vi "ZApproachingPart.vi"() -> ()   [LabVIEW 2014]
uses:
  <vilib>/userdefined/High Color/nirio_resource_hc.ctl
  <vilib>/Instr/_visa.llb/VISA Configure Serial Port (Instr).vi
  <vilib>/FPGAPlugInAG/PCIe-7851R/niLvFpga_Open_PCIe-7851R.vi
  <vilib>/rvi/interface/common/dynamic/niFpgaDynamicAddResources.vi
  <vilib>/Utility/error.llb/Error Cluster From Error Code.vi
  <vilib>/rvi/errors/niLvFpgaAdjustHostInterfaceError.vi
  <vilib>/FPGAPlugInAG/Dynamic/niLvFpga_Close_Dynamic.vi
  <vilib>/rvi/interface/nirviOpenFPGA/nirviOpenFPGA.xnode
  FPGA Bitfiles/FPGATest_FPGATarget_PIZApproaching_ngy2QjQf4ns.lvbitx
  <vilib>/rvi/interface/nirviReadWriteControl/nirviReadWriteControl.xnode
  <vilib>/rvi/interface/nirviCloseFPGA/nirviCloseFPGA.xnode
  FPGA Bitfiles/FPGATest_FPGATarget_PIZWithdraw_iPHi2cM2eR0.lvbitx
  NiFpgaLv.dll
  <vilib>/rvi/interface/Simulation/niFpgaSimulationCallBeginRW.vi
panel:
  out "RoughXYZPosDia":dbl(graph)
  out "RoughXYZErr?":string
  in  "LandingPtRelativeToPIZ/um  Range(0-10)":dbl format="%#_13g"
  out "RoughZPos?":dbl format="%#_13g"
  out "MaxPIZPos":i16
  in  "PIZ":T1
  out "preCurrIndexDia":i16(graph)
  out "preCurrIndex":i16
  out "refCurrIndex":i16
  out "PIZPos":i16
  out "PIZPosDia":i16(graph)
  in  "stop":bool
  in  "AllLoopSleep ms":i32
  in  "thresholdIndex":i32
  in  "RoughXYZ":refnum<visa-resource-name>
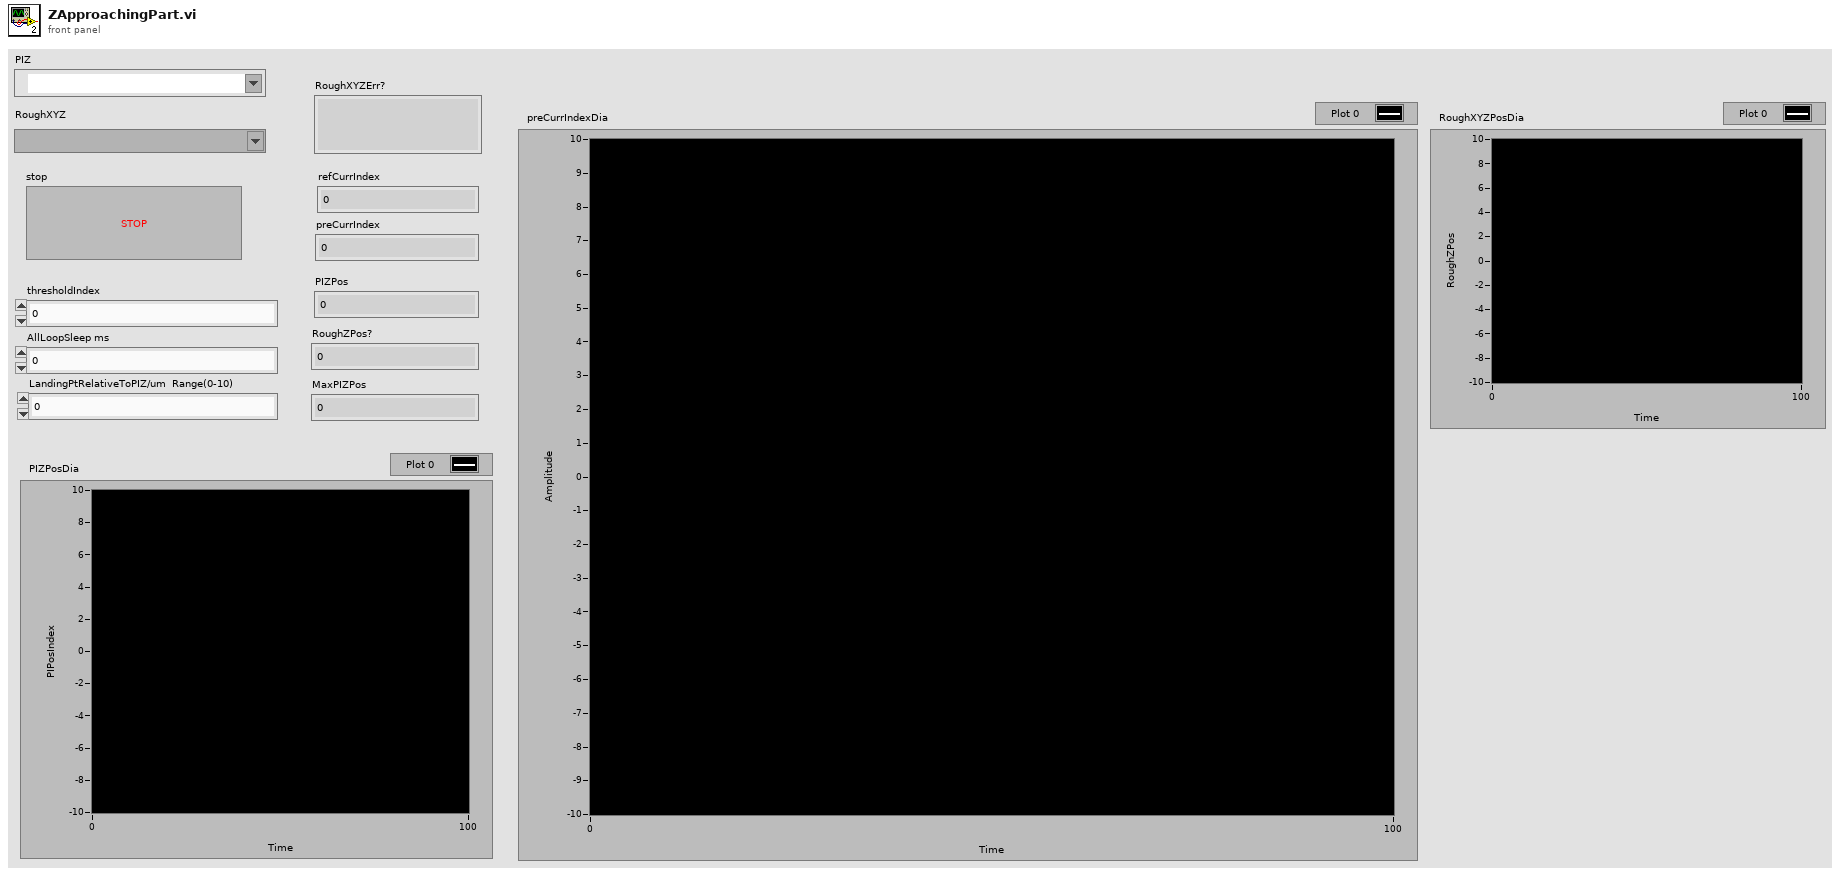
[diagram p1: front panel]
types:
  T1 = typedef "nirio_resource_hc.ctl" = tag
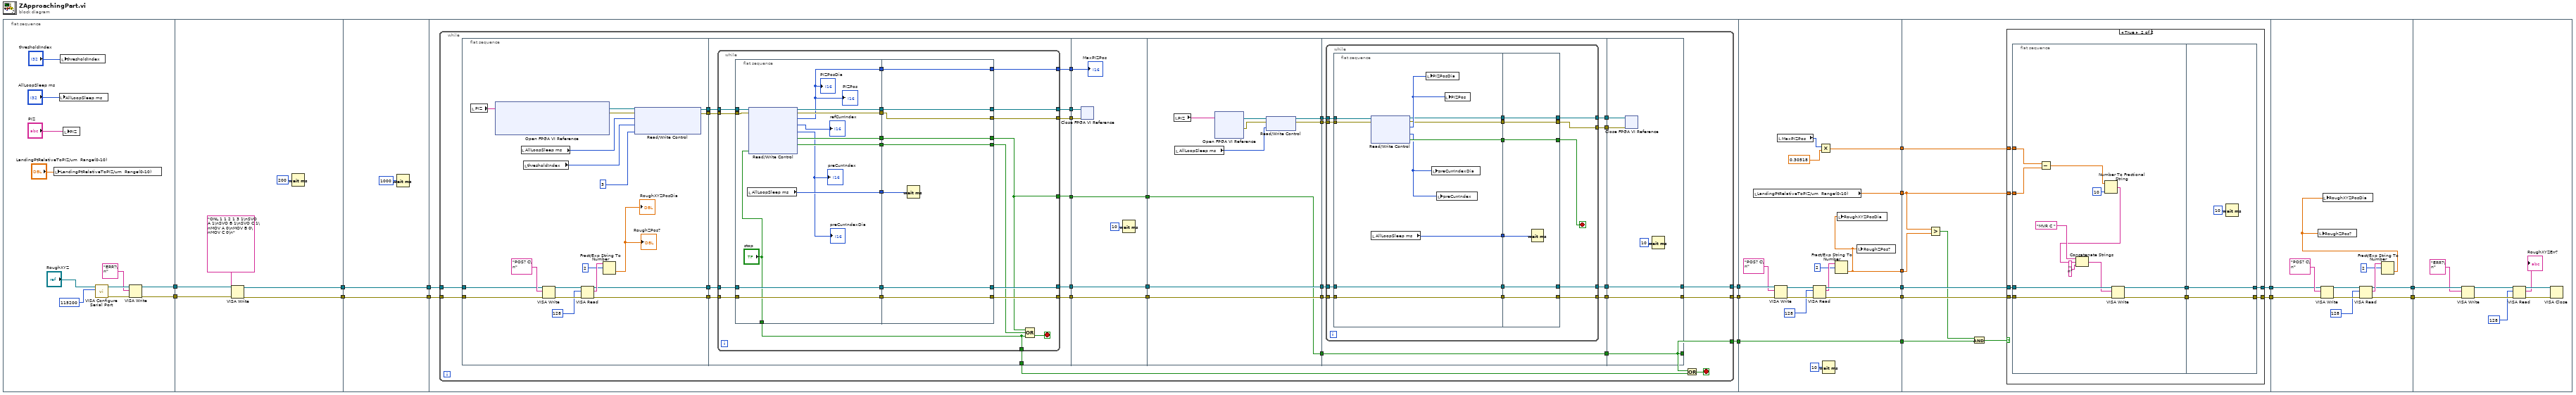
[diagram p0: block diagram]
diagram:
  n1 = flat-sequence {
    tunnel: [w25] -> w19
    tunnel: [w24] -> w18
    tunnel: w19 -> [w36]
    tunnel: w18 -> [w35]
    tunnel: [w33] -> w17
    tunnel: [w32] -> w16
    tunnel: w17 -> [w39]
    tunnel: w16 -> [w38]
    tunnel: [w39] -> w15
    tunnel: [w38] -> w14
    tunnel: w15 -> [w44]
    tunnel: w14 -> [w43]
    tunnel: [w42] -> w13
    tunnel: [w41] -> w11
    tunnel: [w40] -> w10
    tunnel: w13 -> [w225]
    tunnel: [w225] -> w12
    tunnel: w11 -> [w224]
    tunnel: w10 -> [w223]
    tunnel: [w218] -> w9
    tunnel: [w217] -> w8
    tunnel: [w209] -> w7
    tunnel: [w211] -> w6
    tunnel: [w210] -> w5
    tunnel: w12 -> [w231]
    tunnel: w9 -> [w235]
    tunnel: w8 -> [w234]
    tunnel: w7 -> [w229]
    tunnel: w6 -> [w233]
    tunnel: w5 -> [w228]
    tunnel: [w227] -> w4
    tunnel: [w226] -> w3
    tunnel: w4 -> [w265]
    tunnel: w3 -> [w264]
    tunnel: [w263] -> w2
    tunnel: [w262] -> w1
    tunnel: w2 -> [w280]
    tunnel: w1 -> [w279]
    frame #0 {
      n2 = local write "LandingPtRelativeToPIZ/um  Range(0-10)"("LandingPtRelativeToPIZ/um  Range(0-10)") -> ()
      n3 = local write "AllLoopSleep ms"("AllLoopSleep ms") -> ()
      n4 = local write "thresholdIndex"("thresholdIndex") -> ()
      n5 = local write "PIZ"("PIZ") -> ()
      n6 = call-poly "VISA Configure Serial Port"("VISA resource name"="RoughXYZ", "baud rate (9600)"=u32 115200) -> ("VISA resource name out"=w28:refnum<visa-resource-name>, "error out"=w27:errorcluster)  [unwired: 12 in]
      n7 = VISA Write(VISA resource name=w28, write buffer="ERR?\n", error in (no error)=w27) -> (VISA resource name out=w25:refnum<visa-resource-name>, error out=w24:errorcluster)  [unwired: 1 out]
    }
    frame #1 {
      n8 = VISA Write(VISA resource name=w36, write buffer="ONL 1 1 2 1 3 1\nSVO A 1\nSVO B 1\nSVO C 1\nMOV A 0\nMOV B 0\nMOV C 0\n", error in (no error)=w35) -> (VISA resource name out=w33:refnum<visa-resource-name>, error out=w32:errorcluster)  [unwired: 1 out]
      n9 = Wait (ms)(milliseconds to wait=u32 200) -> ()  [unwired: 1 out]
    }
    frame #2 {
      n10 = Wait (ms)(milliseconds to wait=u32 1000) -> ()  [unwired: 1 out]
    }
    frame #3 {
      n11 = while {
        tunnel: w44 -> [w74]
        tunnel: w43 -> [w73]
        tunnel: [w51] -> w42
        tunnel: [w47] -> w41
        tunnel: [w46] -> w40
        stop <- w62 stop-if-true
        n12 = flat-sequence {
          tunnel: w74 -> [w80]
          tunnel: w73 -> [w79]
          tunnel: [w90] -> w72
          tunnel: [w78] -> w71
          tunnel: [w77] -> w70
          tunnel: [w87] -> w57
          tunnel: w72 -> [w104]
          tunnel: w71 -> [w103]
          tunnel: w70 -> [w102]
          tunnel: [w101] -> w69
          tunnel: [w100] -> w68
          tunnel: [w99] -> w67
          tunnel: [w98] -> w66
          tunnel: [w97] -> w45
          tunnel: w57 -> [w96]
          tunnel: [w95] -> w56
          tunnel: [w94] -> w50
          tunnel: w69 -> [w150]
          tunnel: w68 -> [w149]
          tunnel: w67 -> [w151]
          tunnel: w66 -> [w153]
          tunnel: [w151] -> w65
          tunnel: [w150] -> w64
          tunnel: [w149] -> w63
          tunnel: w56 -> [w148]
          tunnel: w50 -> [w147]
          tunnel: w65 -> [w154]
          tunnel: w64 -> [w156]
          tunnel: w63 -> [w155]
          tunnel: [w159] -> w61
          tunnel: [w157] -> w59
          tunnel: [w156] -> w55
          tunnel: [w155] -> w54
          tunnel: [w154] -> w53
          tunnel: w61 -> [w171]
          tunnel: [w170] -> w60
          tunnel: w59 -> [w169]
          tunnel: [w168] -> w58
          tunnel: w55 -> [w167]
          tunnel: w54 -> [w166]
          tunnel: w53 -> [w165]
          tunnel: [w165] -> w52
          tunnel: [w164] -> w49
          tunnel: [w163] -> w48
          tunnel: w60 -> [w208]
          tunnel: w58 -> [w207]
          tunnel: w52 -> [w206]
          tunnel: [w206] -> w51
          tunnel: w49 -> [w204]
          tunnel: w48 -> [w203]
          tunnel: [w204] -> w47
          tunnel: [w203] -> w46
          frame #0 {
            n13 = local read "PIZ"() -> (w89:T1)
            n14 = xnode "Open FPGA VI Reference"("resource name"=w89) -> ("FPGA VI Reference Out"=w93:refnum<k20>, "error out"=w88:errorcluster)  [unwired: 1 in]
            n15 = local read "AllLoopSleep ms"() -> (w92:i32)
            n16 = local read "thresholdIndex"() -> (w91:i32)
            n17 = VISA Write(VISA resource name=w80, write buffer="POS? C\n", error in (no error)=w79) -> (VISA resource name out=w86:refnum<visa-resource-name>, error out=w85:errorcluster)  [unwired: 1 out]
            n18 = VISA Read(VISA resource name=w86, byte count=u32 128, error in (no error)=w85) -> (VISA resource name out=w78:refnum<visa-resource-name>, read buffer=w82:string, error out=w77:errorcluster)  [unwired: 1 out]
            n19 = Fract/Exp String To Number(string=w82, offset=2) -> (number=→"RoughZPos?" →"RoughXYZPosDia":dbl)  [unwired: 2 in, 1 out]
            n20 = xnode "Read/Write Control"("FPGA VI Reference In"=w93, "error in"=w88, "Sleep ms"=w92, "thresholdIndex"=w91, "stepMultiplier / 0.305nm"=i16 3) -> ("FPGA VI Reference Out"=w90:refnum<k20>, "error out"=w87:errorcluster)
          }
          frame #1 {
            n21 = while {
              tunnel: w104 -> [w125]
              tunnel: w103 -> [w122]
              tunnel: w102 -> [w120]
              tunnel: [w115] -> w101
              tunnel: [w114] -> w100
              tunnel: [w113] -> w99
              tunnel: [w111] -> w98
              tunnel: [w110] -> w97
              tunnel: w96 -> [w109]
              tunnel: [w107] -> w95
              tunnel: [w105] -> w94
              stop <- w119 stop-if-true
              n22 = flat-sequence {
                tunnel: w125 -> [w138]
                tunnel: [w137] -> w124
                tunnel: ["stop"] -> w110
                tunnel: [w136] -> w123
                tunnel: w122 -> [w136]
                tunnel: [w135] -> w121
                tunnel: w120 -> [w135]
                tunnel: [w134] -> w118
                tunnel: [w132] -> w117
                tunnel: [w131] -> w116
                tunnel: w109 -> [w128]
                tunnel: [w127] -> w108
                tunnel: [w126] -> w106
                tunnel: w124 -> [w146]
                tunnel: w123 -> [w143]
                tunnel: w121 -> [w142]
                tunnel: w118 -> [w141]
                tunnel: w117 -> [w145]
                tunnel: w116 -> [w144]
                tunnel: [w145] -> w113
                tunnel: [w144] -> w112
                tunnel: [w143] -> w115
                tunnel: [w142] -> w114
                tunnel: [w141] -> w111
                tunnel: w108 -> [w140]
                tunnel: [w140] -> w107
                tunnel: w106 -> [w139]
                tunnel: [w139] -> w105
                frame #0 {
                  n23 = local read "AllLoopSleep ms"() -> (w137:i32)
                  n24 = xnode "Read/Write Control"("FPGA VI Reference In"=w138, "error in"=w128, "stop"="stop") -> ("FPGA VI Reference Out"=w134:refnum<k20>, "error out"=w127:errorcluster, "PIZPos"=w126:i16, "refCurrIndex"=→"refCurrIndex":i16, "preCurrIndex"=→"preCurrIndex" →"preCurrIndexDia":i16, "Approached?"=w132:bool, "NotApproached?"=w131:bool)
                  "PIZPosDia" <- w126
                  "PIZPos" <- w126
                }
                frame #1 {
                  n25 = Wait (ms)(milliseconds to wait=w146) -> ()  [unwired: 1 out]
                }
              }
              n26 = Compound Arithmetic op=OR(w113, w112, w110) -> (w119:bool)
            }
          }
          frame #2 {
            n27 = xnode "Close FPGA VI Reference"("FPGA VI Reference In"=w153, "error in"=w148) -> ()  [unwired: 1 out]
            n28 = Wait (ms)(milliseconds to wait=u32 10) -> ()  [unwired: 1 out]
            "MaxPIZPos" <- w147
          }
          frame #3 {
            n29 = local read "PIZ"() -> (w162:T1)
            n30 = local read "AllLoopSleep ms"() -> (w160:i32)
            n31 = xnode "Open FPGA VI Reference"("resource name"=w162) -> ("FPGA VI Reference Out"=w161:refnum<k20>, "error out"=w158:errorcluster)  [unwired: 1 in]
            n32 = xnode "Read/Write Control"("FPGA VI Reference In"=w161, "error in"=w158, "Sleep ms"=w160) -> ("FPGA VI Reference Out"=w159:refnum<k20>, "error out"=w157:errorcluster)
          }
          frame #4 {
            n33 = while {
              tunnel: w171 -> [w186]
              tunnel: [w181] -> w170
              tunnel: w169 -> [w180]
              tunnel: [w178] -> w168
              tunnel: w167 -> [w177]
              tunnel: w166 -> [w176]
              tunnel: [w173] -> w164
              tunnel: [w172] -> w163
              stop <- w184 stop-if-true
              n34 = flat-sequence {
                tunnel: w186 -> [w196]
                tunnel: [w195] -> w185
                tunnel: [w192] -> w183
                tunnel: [w191] -> w182
                tunnel: w180 -> [w190]
                tunnel: [w189] -> w179
                tunnel: w177 -> [w188]
                tunnel: w176 -> [w187]
                tunnel: [w188] -> w175
                tunnel: [w187] -> w174
                tunnel: w185 -> [w202]
                tunnel: [w202] -> w184
                tunnel: w183 -> [w201]
                tunnel: w182 -> [w200]
                tunnel: [w200] -> w181
                tunnel: [w199] -> w178
                tunnel: w179 -> [w199]
                tunnel: [w198] -> w173
                tunnel: w175 -> [w198]
                tunnel: [w197] -> w172
                tunnel: w174 -> [w197]
                frame #0 {
                  n35 = xnode "Read/Write Control"("FPGA VI Reference In"=w196, "error in"=w190) -> ("FPGA VI Reference Out"=w191:refnum<k20>, "error out"=w189:errorcluster, "PIZPos?"=w194:i16, "preCurrIndex"=w193:i16, "Withdrawn?"=w195:bool)
                  n36 = local read "AllLoopSleep ms"() -> (w192:i32)
                  n37 = local write "PIZPosDia"(w194) -> ()
                  n38 = local write "preCurrIndexDia"(w193) -> ()
                  n39 = local write "preCurrIndex"(w193) -> ()
                  n40 = local write "PIZPos"(w194) -> ()
                }
                frame #1 {
                  n41 = Wait (ms)(milliseconds to wait=w201) -> ()  [unwired: 1 out]
                }
              }
            }
          }
          frame #5 {
            n42 = xnode "Close FPGA VI Reference"("FPGA VI Reference In"=w208, "error in"=w207) -> ()  [unwired: 1 out]
            n43 = Wait (ms)(milliseconds to wait=u32 10) -> ()  [unwired: 1 out]
          }
        }
        n44 = Or(x=w51, y=w45) -> (x .or. y?=w62:bool)
      }
    }
    frame #4 {
      n45 = local read "LandingPtRelativeToPIZ/um  Range(0-10)"() -> (w210:dbl)
      n46 = VISA Write(VISA resource name=w224, write buffer="POS? C\n", error in (no error)=w223) -> (VISA resource name out=w222:refnum<visa-resource-name>, error out=w221:errorcluster)  [unwired: 1 out]
      n47 = local read "MaxPIZPos"() -> (w213:i16)
      n48 = VISA Read(VISA resource name=w222, byte count=u32 128, error in (no error)=w221) -> (VISA resource name out=w218:refnum<visa-resource-name>, read buffer=w216:string, error out=w217:errorcluster)  [unwired: 1 out]
      n49 = Multiply(x=w213, y=0.30518) -> (x*y=w211:dbl)
      n50 = Wait (ms)(milliseconds to wait=u32 10) -> ()  [unwired: 1 out]
      n51 = Fract/Exp String To Number(string=w216, offset=2) -> (number=w209:dbl)  [unwired: 2 in, 1 out]
      n52 = local write "RoughXYZPosDia"(w209) -> ()
      n53 = local write "RoughZPos?"(w209) -> ()
    }
    frame #5 {
      n54 = Greater?(x=w228, y=w229) -> (0:w230:bool)
      n55 = And(x=w230, y=w231) -> (x .and. y?=w232:bool)
      n56 = case shown="True" w232 {
        tunnel: w235 -> [w237 w245]
        tunnel: w234 -> [w236 w244]
        tunnel: w233 -> [_ w242]
        tunnel: w228 -> [_ w243]
        tunnel: [w237 w239] -> w227
        tunnel: [w236 w238] -> w226
        frame False {
        }
        frame True {
          n57 = flat-sequence {
            tunnel: w245 -> [w255]
            tunnel: w244 -> [w254]
            tunnel: w243 -> [w256]
            tunnel: w242 -> [w257]
            tunnel: [w247] -> w241
            tunnel: [w246] -> w240
            tunnel: w241 -> [w259]
            tunnel: w240 -> [w258]
            tunnel: [w259] -> w239
            tunnel: [w258] -> w238
            frame #0 {
              n58 = Subtract(x=w257, y=w256) -> (x-y=w252:dbl)
              n59 = Number To Fractional String(number=w252, precision (6)=i16 10) -> (F-format string=w250:string)  [unwired: 2 in]
              n60 = Concatenate Strings("MVR C " ("string"), w250, "\n" ("string")) -> (w248:string)
              n61 = VISA Write(VISA resource name=w255, write buffer=w248, error in (no error)=w254) -> (VISA resource name out=w247:refnum<visa-resource-name>, error out=w246:errorcluster)  [unwired: 1 out]
            }
            frame #1 {
              n62 = Wait (ms)(milliseconds to wait=u32 10) -> ()  [unwired: 1 out]
            }
          }
        }
      }
    }
    frame #6 {
      n63 = VISA Write(VISA resource name=w265, write buffer="POS? C\n", error in (no error)=w264) -> (VISA resource name out=w271:refnum<visa-resource-name>, error out=w270:errorcluster)  [unwired: 1 out]
      n64 = VISA Read(VISA resource name=w271, byte count=u32 128, error in (no error)=w270) -> (VISA resource name out=w263:refnum<visa-resource-name>, read buffer=w267:string, error out=w262:errorcluster)  [unwired: 1 out]
      n65 = Fract/Exp String To Number(string=w267, offset=2) -> (number=w261:dbl)  [unwired: 2 in, 1 out]
      n66 = local write "RoughZPos?"(w261) -> ()
      n67 = local write "RoughXYZPosDia"(w261) -> ()
    }
    frame #7 {
      n68 = VISA Write(VISA resource name=w280, write buffer="ERR?\n", error in (no error)=w279) -> (VISA resource name out=w277:refnum<visa-resource-name>, error out=w276:errorcluster)  [unwired: 1 out]
      n69 = VISA Read(VISA resource name=w277, byte count=u32 128, error in (no error)=w276) -> (VISA resource name out=w275:refnum<visa-resource-name>, read buffer=→"RoughXYZErr?":string, error out=w274:errorcluster)  [unwired: 1 out]
      n70 = VISA Close(VISA resource name=w275, error in (no error)=w274) -> ()  [unwired: 1 out]
    }
  }
